vi "配置读取.vi"(8 "error in (no error)":errorcluster caption="错误输入（无错误）", 11 "TimingControl 输入":refnum<class "TimingControl.lvclass">) -> (0 "error out":errorcluster caption="错误输出", 3 "TimingControl 输出":refnum<class "TimingControl.lvclass">)   [LabVIEW 2016, in "ZKTimingControl.lvlib" / "TimingControl.lvclass"]
uses:
  TimingControl.lvclass
  TimingControl.lvclass/TimingControl.ctl
  <vilib>/Utility/xml.llb/Read From XML File(string).vi
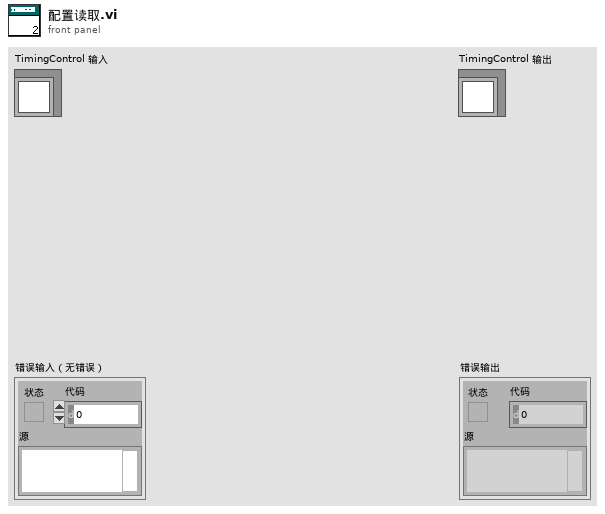
[diagram p1: front panel]
types:
  T1 = typedef "ZKTimingControl.lvlib/TimingControl.lvclass/State Data.ctl" = cluster{"仪器时间":timestamp, "仪器运行状态":bool, "配置文件路径":path, "测量参数":T2, "测试状态":cluster{"启动时间":timestamp, "结束时间":timestamp, "启动次数":dbl}, "配置信息":T3}
  T2 = typedef "ZKTimingControl.lvlib/TimingControl.lvclass/测量参数.ctl" = cluster{"氨氮":bool, "总磷":bool, "总氮":bool, "CODMn":bool, "CODCr":bool}
  T3 = typedef "ZKTimingControl.lvlib/TimingControl.lvclass/配置信息.ctl" = cluster{"每周启动":T4, "每月启动":T5, "周期模式":T6, "测量参数":T2, "定点周期":T7, "间隔启动":T9, "配置时间":timestamp}
  T4 = typedef "ZKTimingControl.lvlib/TimingControl.lvclass/每周启动.ctl" = enum16{"关闭", "周日", "周一", "周二", "周三", "周四", "周五", "周六"}
  T5 = typedef "ZKTimingControl.lvlib/TimingControl.lvclass/每月启动.ctl" = enum16{"关闭", "1号", "2号", "3号", "4号", "5号", "6号", "7号", "8号", "9号", "10号", "11号", "12号", "13号", "14号", "15号", "16号", "17号", "18号", "19号", "20号", "21号", "22号", "23号", "24号", "25号", "26号", "27号", "28号", "29号", "30号", "31号"}
  T6 = typedef "ZKTimingControl.lvlib/TimingControl.lvclass/周期模式设置.ctl" = enum16{"不启用", "定点模式", "间隔模式"}
  T7 = typedef "ZKTimingControl.lvlib/TimingControl.lvclass/定点周期设置.ctl" = cluster{"启动命令":T8, "启动命令 2":T8, "启动命令 3":T8, "启动命令 4":T8, "启动命令 5":T8, "启动命令 6":T8, "启动命令 7":T8, "启动命令 8":T8, "启动命令 9":T8, "启动命令 10":T8, "启动命令 11":T8, "启动命令 12":T8, "启动命令 13":T8, "启动命令 14":T8, "启动命令 15":T8, "启动命令 16":T8, "启动命令 17":T8, "启动命令 18":T8, "启动命令 19":T8, "启动命令 20":T8, "启动命令 21":T8, "启动命令 22":T8, "启动命令 23":T8, "启动命令 24":T8}
  T8 = typedef "ZKTimingControl.lvlib/TimingControl.lvclass/启动命令选择.ctl" = enum16{"", "加标回收（启动采配水）", "加标回收（不启动采配水）", "水样测试（启动采配水）", "水样测试（不启动采配水）", "平行样测试（启动采配水）", "平行样测试（不启动采配水）", "集成干预测试"}
  T9 = typedef "ZKTimingControl.lvlib/TimingControl.lvclass/间隔启动设置.ctl" = cluster{"启动命令":T8, "启动间隔":dbl, "启动次数":i32}
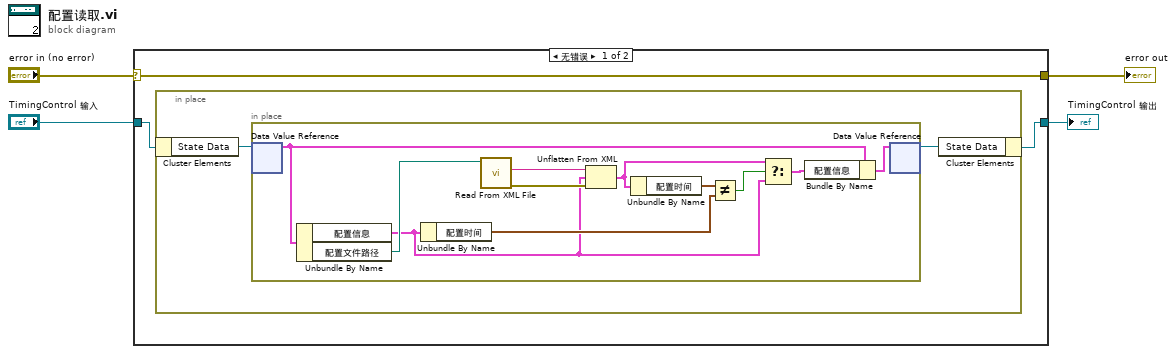
[diagram p0: block diagram]
diagram:
  n1 = case shown="无错误" "error in (no error)" {
    selector: "error in (no error)" -> [w7 w22]
    tunnel: [w7 w22] -> w3
    tunnel: [w5 w21] -> w1
    tunnel: "TimingControl 输入" -> [w6 w21]
    frame No Error {
      n2 = in-place {
        n3 = in-place-cluster #1(w6) -> ("State Data"=w9:refnum<data-value>)
        n4 = in-place {
          n5 = in-place-dvr #2(w9) -> (w19:T1)  [unwired: 1 out]
          n6 = Unbundle By Name(w19) -> ("配置信息"=w11:T3, "配置文件路径"=w18:path)
          n7 = Unbundle By Name(w11) -> ("配置时间"=w14:timestamp)
          n8 = call-poly <vilib>:"Read From XML File.vi"("XML File Path"=w18) -> ("error out"=w17:errorcluster, "XML Elements"=w16:string)  [unwired: 8 in, 1 out]
          n9 = Unflatten From XML(xml string=w16, type=w11, error in (no error)=w17) -> (value=w12:T3)  [unwired: 1 out]
          n10 = Unbundle By Name(w12) -> ("配置时间"=w15:timestamp)
          n11 = Not Equal?(x=w15, y=w14) -> (x != y?=w13:bool)
          n12 = Select(t=w12, s=w13, f=w11) -> (s? t:f=w10:T3)
          n13 = Bundle By Name(cluster=w19, "配置信息"=w10) -> (w20:T1)
          n14 = in-place-dvr #2(w20) -> (w8:refnum<data-value>)  [unwired: 1 out]
        }
        n15 = in-place-cluster #1("State Data"=w8) -> (w5:refnum<class "TimingControl.lvclass">)
      }
    }
    frame Error {
    }
  }
  "error out" <- w3
  "TimingControl 输出" <- w1
